vi "Counter Acquisition Setup.vi"(11 "Count Edges Data":T1) -> (0 "error out":errorcluster, 3 "Refnum out":refnum<k21>)   [LabVIEW 2021]
doc: "This VI receives the cluster data necessary to setup and start the DAQmx counter input data acquisition."
uses:
  <vilib>/DAQmx/create/channels.llb/DAQmx Create Channel (CI-Count Edges).vi
  <resource>/objmgr/daqmx.rc
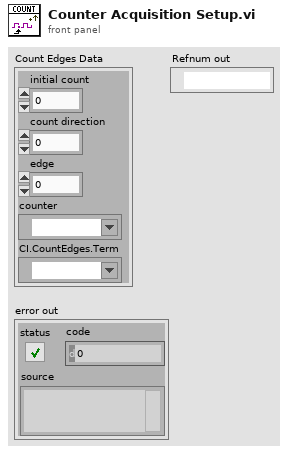
[diagram p1: front panel]
types:
  T1 = cluster{"initial count":u32, "count direction":i32, "edge":i32, "counter":tag, "CI.CountEdges.Term":tag}
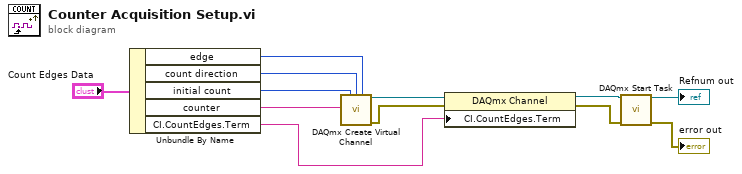
[diagram p0: block diagram]
diagram:
  n1 = Unbundle By Name("Count Edges Data") -> ("edge"=w10:i32, "count direction"=w9:i32, "initial count"=w8:u32, "counter"=w11:tag, "CI.CountEdges.Term"=w12:tag)
  n2 = call-poly <vilib>:"DAQmx Create Virtual Channel.vi"("initial count"=w8, "count direction"=w9, "edge"=w10, "counter"=w11) -> ("task out"=w2:refnum<k21>, "error out"=w4:errorcluster)  [unwired: 10 in]
  n3 = property class="DAQmx Channel"(reference=w2, error in=w4, "CI.CountEdges.Term"=w12) -> (reference out=w3:refnum<k21>, error out=w5:errorcluster)
  n4 = call <vilib>:"DAQmx Start Task.vi"("task/channels in"=w3, "error in"=w5) -> ("task out"=→"Refnum out":refnum<k21>, "error out"=→"error out":errorcluster)  [unwired: 12 in]
